vi "UI Main.vi"() -> ()   [LabVIEW 2013]
uses:
  controls/Control Configuration.ctl
  controls/Custom Controller Inputs.ctl
  controls/UI Data.ctl
  controls/All FPGA Configuration Values.ctl
  controls/FPGA State.ctl
  controls/Raw Values.ctl
  Globals/Global - All UI Loop Stop.vi
  Globals/Global - UI Stream and Variable Connections.vi
  Globals/Global - Configuration Options.vi
  support/User Event - Stop/User Event - Stop.lvlib
  support/Message Queue/Message Queue.lvlib
  <vilib>/Analysis/NI_AALBase.lvlib
panel:
  out "Connected? 2":bool=TRUE
  in  "Switch to Safe State":bool
  in  "Exit":bool
  out "System Status":string="\n5/12/2014 3:31:58 PM: UI Error -314220 - Read Single Element from Stream in UI - Read Stream from RT.vi->UI Main.vi\n5/12/2014 3:31:58 PM: UI Error -314220 - Read Single Element from Stream in UI - Read Stream from RT.vi->UI Main.vi\n5/12/2014 3:31:58 PM: UI Error -314220 - Read Single Element from Stream in UI - Read Stream from RT.vi->UI Main.vi\n5/12/2014 3:31:58 PM: UI Error -314220 - Read Single Element from Stream in UI - Read Stream from RT.vi->UI Main.vi\n5/12/2014 3:31:58 PM: UI Error -314220 - Read Single Element from Stream in UI - Read Stream from RT.vi->UI Main.vi\n5/12/2014 3:31:58 PM: UI Error -314220 - Read Single Element from Stream in UI - Read Stream from RT.vi->UI Main.vi\n5/12/2014 3:31:58 PM: UI Error -314220 - Read Single Element from Stream in UI - Read Stream from RT.vi->UI Main.vi\n5/12/2014 3:31:58 PM: UI Error -314220 - Read Single Element from Stream in UI - Read Stream from RT.vi->UI Main.vi\n5/12/2014 3:31:58 PM: UI Error -314220 - Read Single Element from Stream in UI - Read Stream from RT.vi->UI Main.vi\n5/12/2014 3:31:58 PM: UI Error -314220 - Read Single Element from Stream in UI - Read Stream from RT.vi->UI Main.vi\n5/12/2014 3:31:58 PM: UI Error -314220 - Read Single Element from Stream in UI - Read Stream from RT.vi->UI Main.vi\n5/12/2014 3:31:58 PM: UI Error -314220 - Read Single Element from Stream in UI - Read Stream from RT.vi->UI Main.vi\n5/12/2014 3:31:58 PM: UI Error -314220 - Read Single Element from Stream in UI - Read Stream from RT.vi->UI Main.vi\n5/12/2014 3:31:58 PM: UI Error -314220 - Read Single Element from Stream in UI - Read Stream from RT.vi->UI Main.vi\n5/12/2014 3:31:58 PM: UI Error -314220 - Read Single Element from Stream in UI - Read Stream from RT.vi->UI Main.vi\n5/12/2014 3:31:58 PM: UI Error -314220 - Read Single Element from Stream in UI - Read Stream from RT.vi->UI Main.vi\n5/12/2014 3:31:58 PM: UI Error -314220 - Write Single Element to Stream in UI Main.vi\n5/12/2014 3:31:36 PM: UI Error -314004 - Create Network Stream Writer Endpoint in UI - Initiate Connection.vi->UI Main.vi\n5/6/2014 11:02:04 PM: UI Error -314220 - Write Single Element to Stream in UI Main.vi"
  out "Current FPGA Control Mode":u16(ring)=2 items=["Safe State", "Manual", "Control (PID)"]
  in  "Settings Tab":T1(tab)
  in  "Control period (ticks)":u32=40000
  in  "Auto tare":bool
  in  "Channel 3 Setpoint":fxp<+/-,16,5>
  in  "Channel 2 Setpoint":fxp<+/-,16,5>
  in  "Channel 1 Setpoint":fxp<+/-,20,7>=7.0
  in  "Channel 0 Setpoint":fxp<+/-,20,7>
  in  "Update Control Configuration":bool
  in  "Control Configurations":T2[](array[typedef])=[{"PID Gains"={"proportional gain (Kc)"=55.0, "integral gain (Kc*Ts/Ti)"=0.0, "derivative gain (Kc*Td/Ts)"=0.0}, "Output Range"={"output high"=50.0, "output low"=-50.0}}, {"PID Gains"={"proportional gain (Kc)"=0.0, "integral gain (Kc*Ts/Ti)"=0.0, "derivative gain (Kc*Td/Ts)"=0.0}, "Output Range"={"output high"=10.0, "output low"=-10.0}}, {"PID Gains"={"proportional gain (Kc)"=0.0, "integral gain (Kc*Ts/Ti)"=0.0, "derivative gain (Kc*Td/Ts)"=0.0}, "Output Range"={"output high"=10.0, "output low"=-10.0}}, {"PID Gains"={"proportional gain (Kc)"=0.0, "integral gain (Kc*Ts/Ti)"=0.0, "derivative gain (Kc*Td/Ts)"=0.0}, "Output Range"={"output high"=10.0, "output low"=-10.0}}]
  in  "Run Control":bool
  in  "Stop Control":bool
  in  "Custom Controller Inputs":T3={"Other Controller Gains"={"Position Control Kp"=0.0, "Virtual Spring Constant (N/m)"=1000.0, "Offset weight (N)"=0.0, "Fthresh (N)"=1.0, "Var2"=0.0}}
  out "Offset (N)":fxp<+/-,16,8>
  in  "Channel 3 Manual Value":fxp<+/-,16,5>
  in  "Channel 2 Manual Value":fxp<+/-,16,5>
  in  "Channel 1 Manual Value":fxp<+/-,16,5>
  in  "Channel 0 Manual Value":fxp<+/-,16,5>
  in  "Run Manual":bool
  in  "Stop Manual":bool
  in  "Retain data":bool
  out "F std":dbl format="%#_4g"
  out "F avg":dbl format="%#_4g"
  in  "Clear Button":bool
  in  "Pause Button":bool
  in  "Save As Button":bool
  in  "Display frequency (Hz)":dbl=200.0 min=1.0 step=1.0
  out "Inputs (mV or V)":cluster{dbl[], dbl[]}[](graph)
  in  "Number of points":i32=1000 min=1 max=500000
  out "Force (N)":cluster{dbl[], dbl[]}(graph)
  out "V*":cluster{dbl[], dbl[]}(graph)
  out "Position (mm)":cluster{dbl[], dbl[]}(graph)
  out "Control loop frequency (Hz)":u32=40006
  out "Actual Loop Period (ticks)":u32=40006
  out "Largest Contiguous Memory (bytes)":dbl(graph)=60041648.0
  out "CPU Usage (%)":dbl(graph)=8.354955497028612
  out "Connected?":bool=TRUE
  in  "Connect to Controller":bool
  in  "Controller Address":string="169.254.66.100"
  # "LabVIEW FPGA Control on CompactRIO"
  # "Connection Settings"
  # "Force Command (N)"
  # "Position Command (mm)"
  # "Current Command (Testing)"
  # "Control period and setpoint changes are sent to the target automatically."
  # "Control Configuration changes are sent to the target when you click \"Update Control Configurations\"."
  # "Not used"
  # "Not used"
  # "Not used"
  # "F ="
  # "+/-"
  # "N"
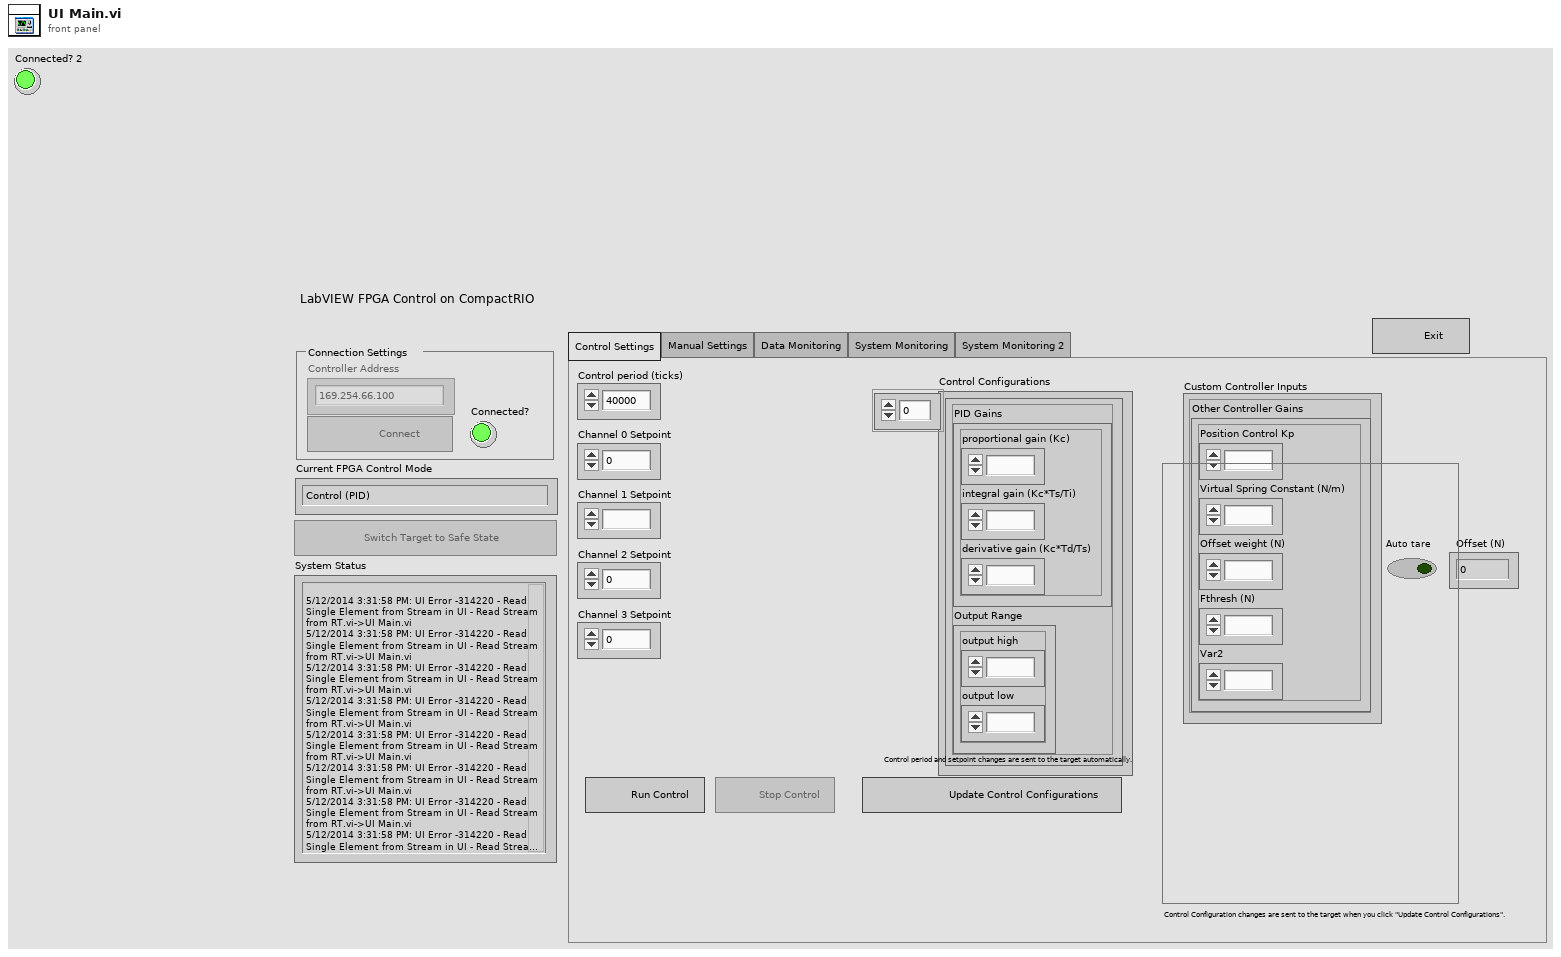
[diagram p1: front panel]
types:
  T1 = enum32{"Control Settings", "Manual Settings", "Data Monitoring", "System Monitoring", "System Monitoring 2"}
  T2 = typedef "Control Configuration.ctl" = cluster{"PID Gains":cluster{"proportional gain (Kc)":fxp<+/-,16,8>, "integral gain (Kc*Ts/Ti)":fxp<+/-,16,8>, "derivative gain (Kc*Td/Ts)":fxp<+/-,16,8>}, "Output Range":cluster{"output high":fxp<+/-,16,7>, "output low":fxp<+/-,16,7>}}
  T3 = typedef "Custom Controller Inputs.ctl" = cluster{"Other Controller Gains":cluster{"Position Control Kp":fxp<+/-,16,8>, "Virtual Spring Constant (N/m)":fxp<+,16,12>, "Offset weight (N)":fxp<+/-,16,8>, "Fthresh (N)":fxp<+/-,16,5>, "Var2":fxp<+/-,16,5>}}
  T4 = typedef "UI Data.ctl" = cluster{"Switch to Safe State Ref":refnum<vi>, "Run Manual Ref":refnum<vi>, "Stop Manual Ref":refnum<vi>, "Run Control Ref":refnum<vi>, "Stop Control Ref":refnum<vi>, "Update Control Configurations Ref":refnum<vi>, "Ch 0 Setpoint Ref":refnum<vi>, "Ch 1 Setpoint Ref":refnum<vi>, "Ch 2 Setpoint Ref":refnum<vi>, "Ch 3 Setpoint Ref":refnum<vi>, "Ch 0 Manual Ref":refnum<vi>, "Ch 1 Manual Ref":refnum<vi>, "Ch 2 Manual Ref":refnum<vi>, "Ch 3 Manual Ref":refnum<vi>, "Control Configurations Ref":refnum<vi>, "Custom Controller Cluster Ref":refnum<vi>, "Control period (ticks) Ref":refnum<vi>}
  T5 = typedef "Message Queue.lvlib/All Message Queues.ctl" = cluster{"UI":refnum<queue>}
  T6 = enum16{"open", "replace", "create", "open or create", "replace or create", "replace or create with confirmation"}
  T7 = cluster{"Channel 0 Setpoint":fxp<+/-,20,7>, "Channel 1 Setpoint":fxp<+/-,20,7>, "Channel 2 Setpoint":fxp<+/-,16,5>, "Channel 3 Setpoint":fxp<+/-,16,5>}
  T8 = cluster{"Channel 0 Manual Value":fxp<+/-,16,5>, "Channel 1 Manual Value":fxp<+/-,16,5>, "Channel 2 Manual Value":fxp<+/-,16,5>, "Channel 3 Manual Value":fxp<+/-,16,5>}
  T9 = typedef "Variable References.ctl" = cluster{"CPU Usage":refnum<k21>, "Contiguous Memory":refnum<k21>, "Input Values":refnum<k21>, "Output Values":refnum<k21>, "FPGA Mode":refnum<k21>, "Actual Loop Period":refnum<k21>}
  T10 = typedef "Raw Values.ctl" = cluster{"Channel 0":fxp<+/-,20,7>, "Channel 1":fxp<+/-,20,7>, "Channel 2":fxp<+/-,20,7>, "Channel 3":fxp<+/-,20,14>}
  T11 = cluster{"Channel 0":dbl, "Channel 1":dbl, "Channel 2":dbl, "Channel 3":dbl}
  T12 = cluster{"Message":string, "Message Data":variant}
  T13 = typedef "All FPGA Configuration Values.ctl" = cluster{"FPGA State":T14, "Manual Values":T10, "Setpoints":T10, "Control Configurations":T2[]}
  T14 = typedef "FPGA State.ctl" = enum16{"Safe State", "Manual", "Control (PID)"}
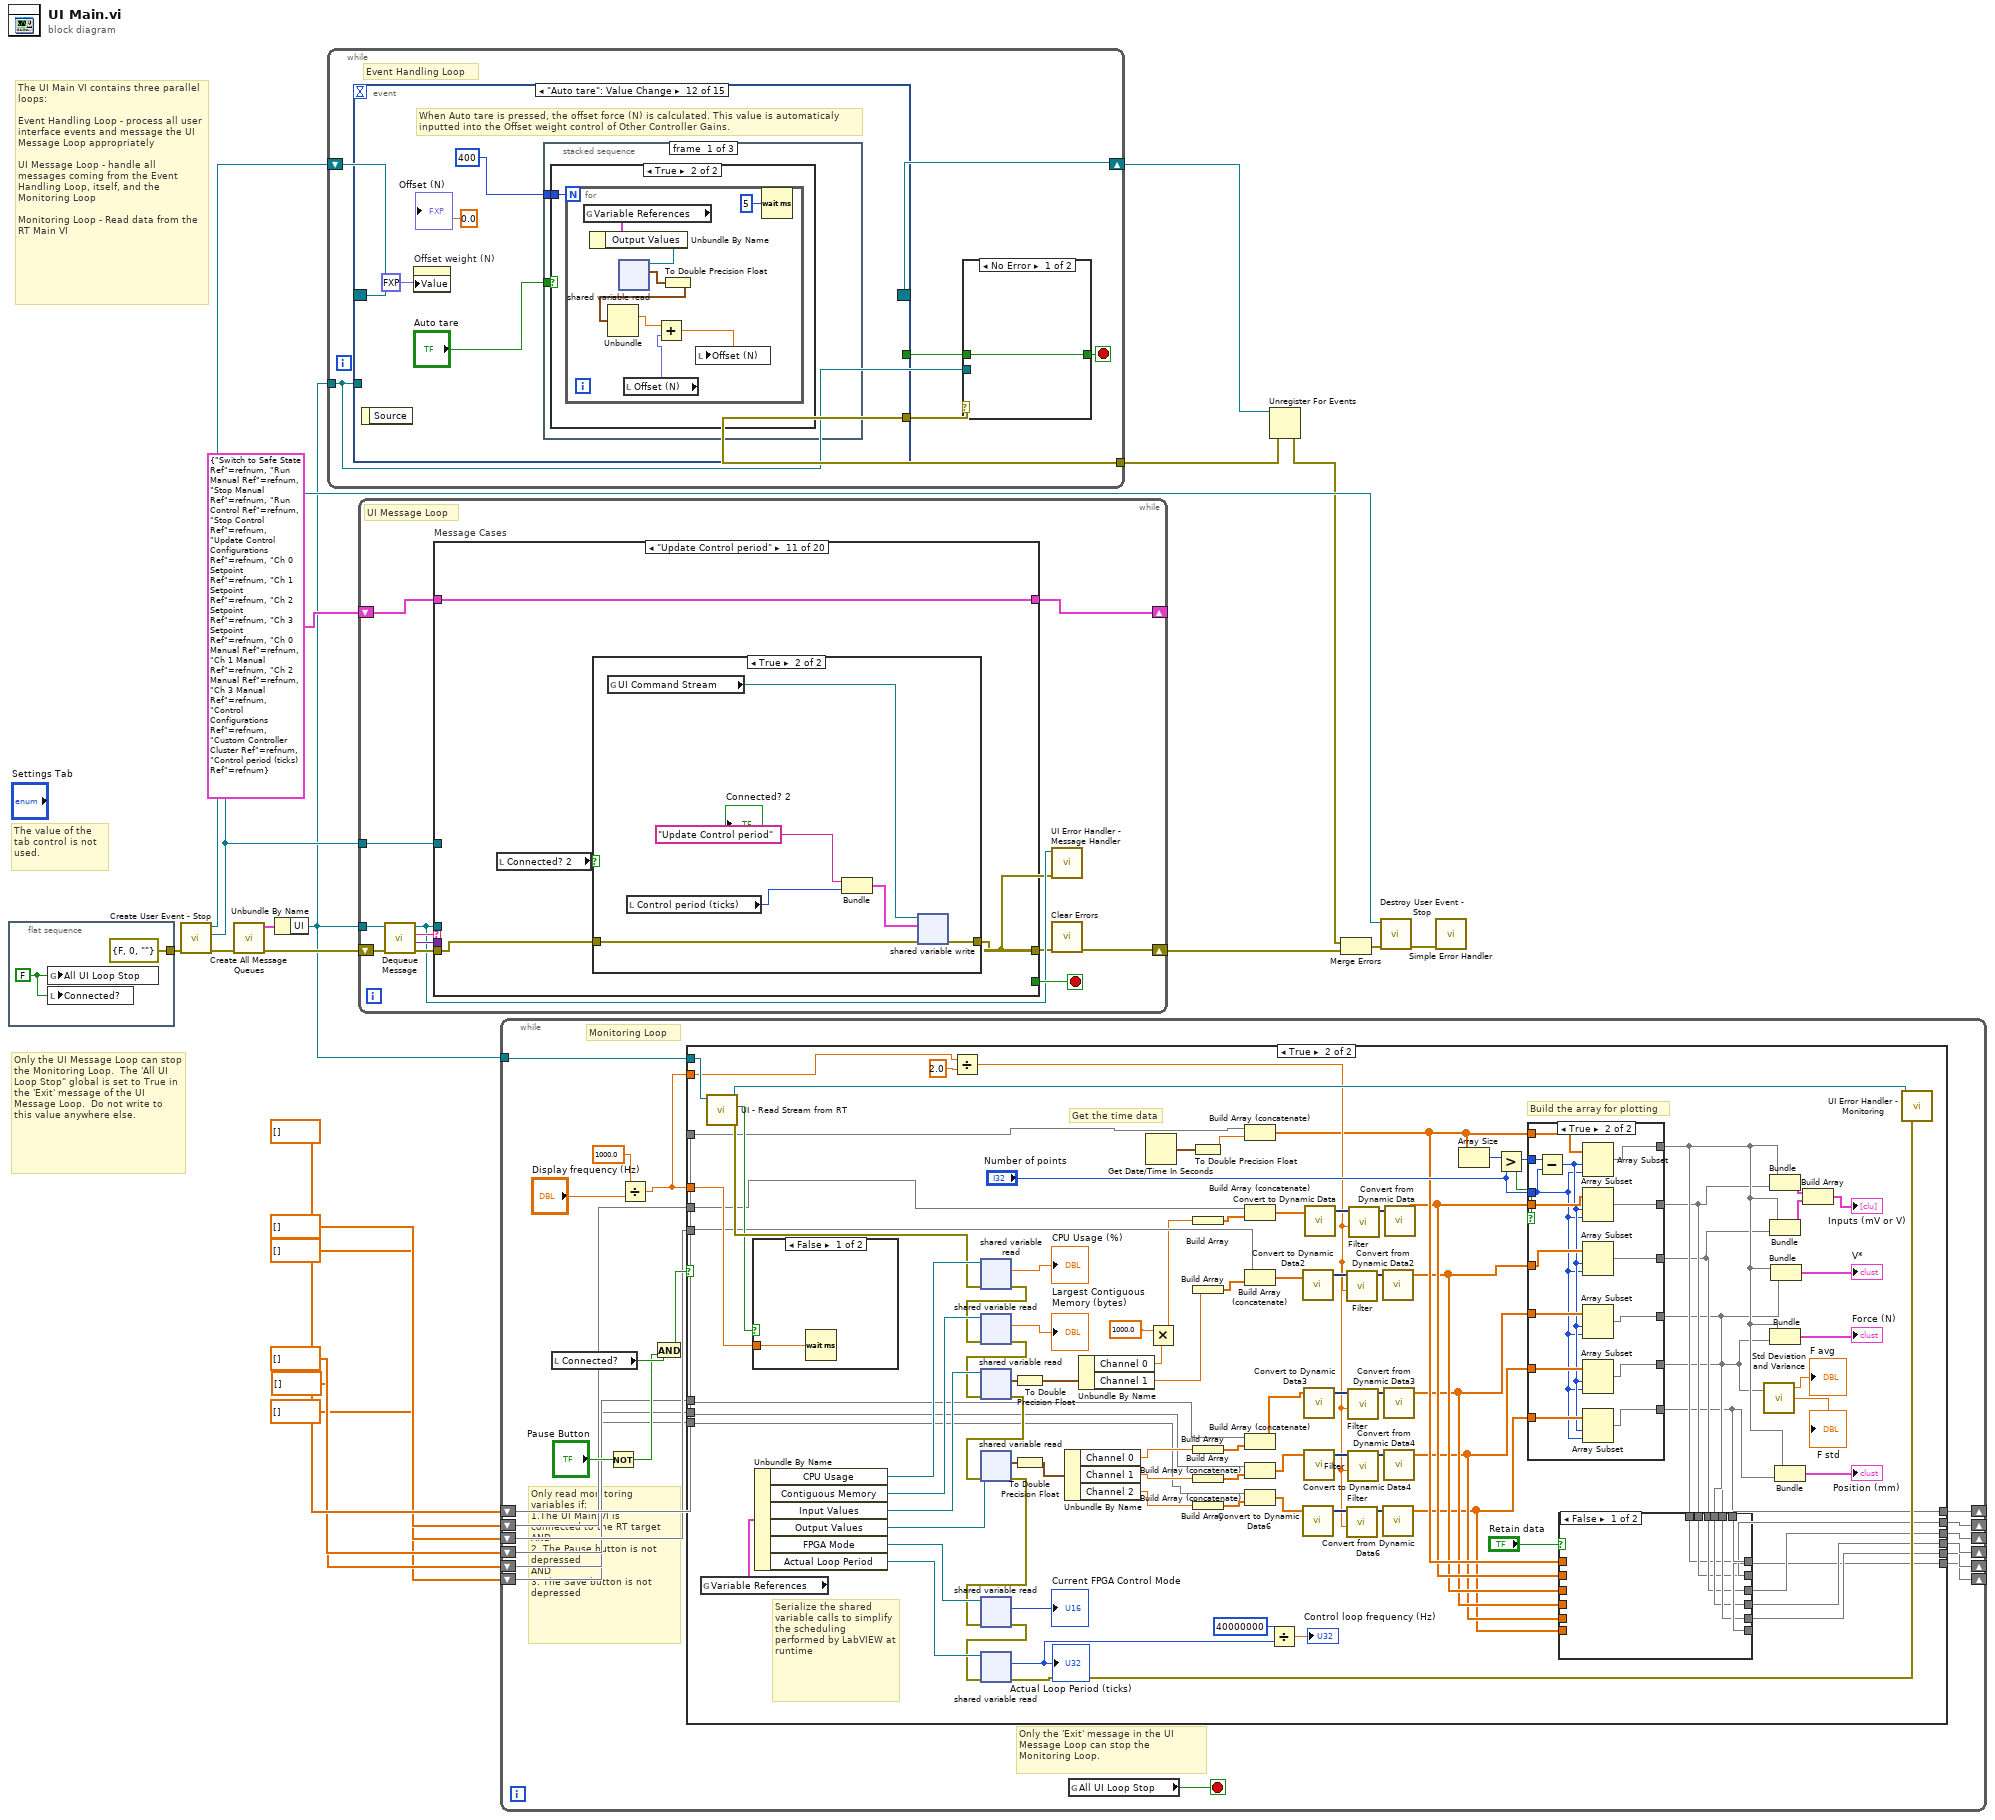
[diagram p0: block diagram]
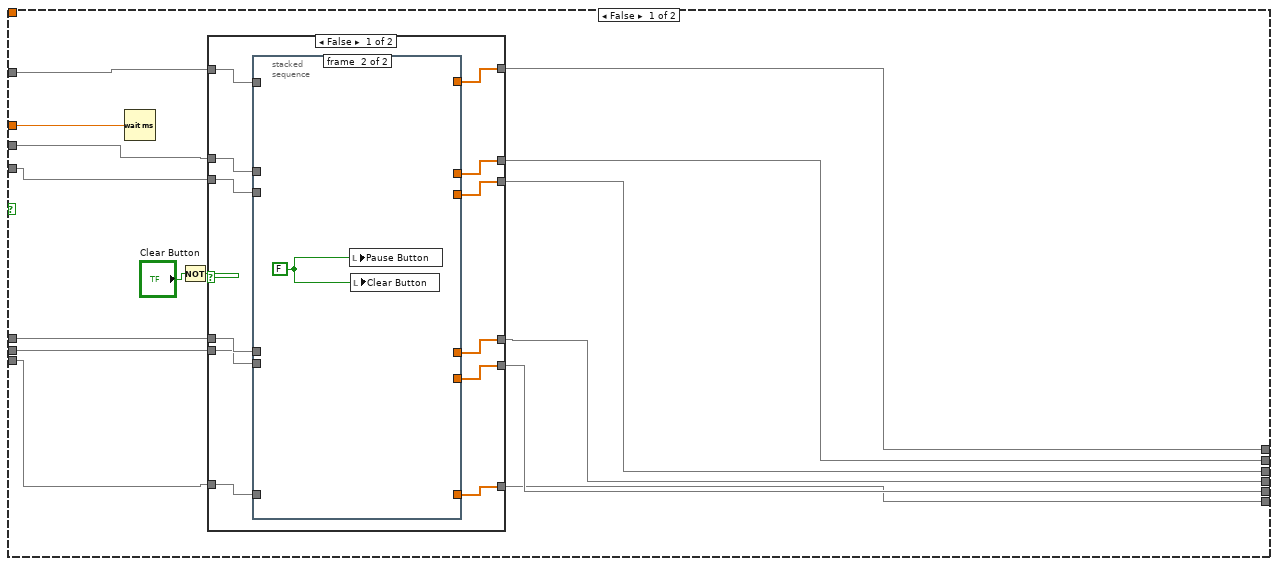
[diagram p2: hidden frame]
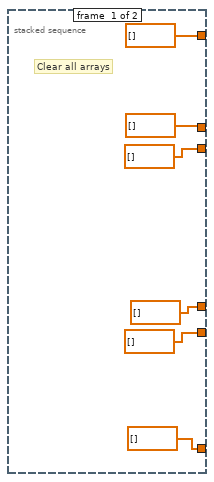
[diagram p3: hidden frame]
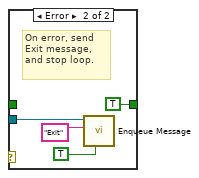
[diagram p8: hidden frame]
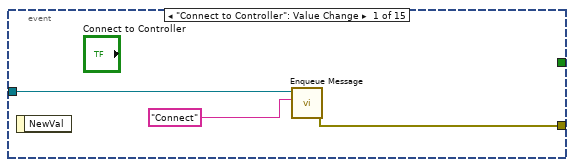
[diagram p9: hidden frame]
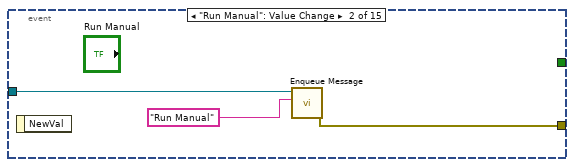
[diagram p10: hidden frame]
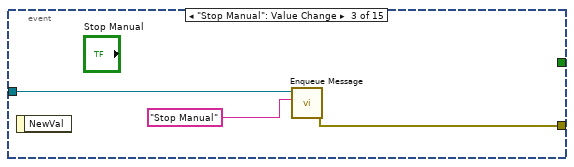
[diagram p11: hidden frame]
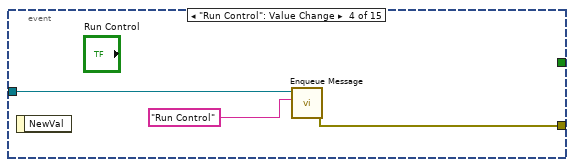
[diagram p12: hidden frame]
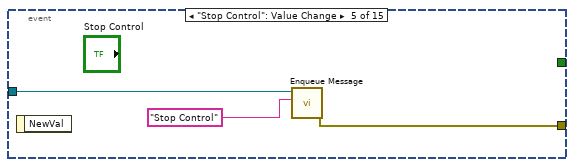
[diagram p13: hidden frame]
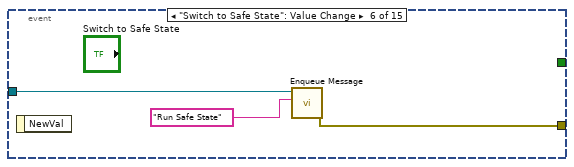
[diagram p14: hidden frame]
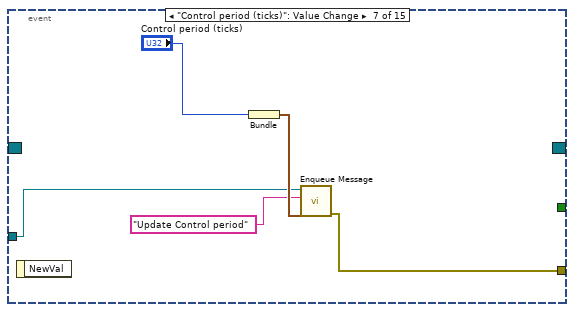
[diagram p15: hidden frame]
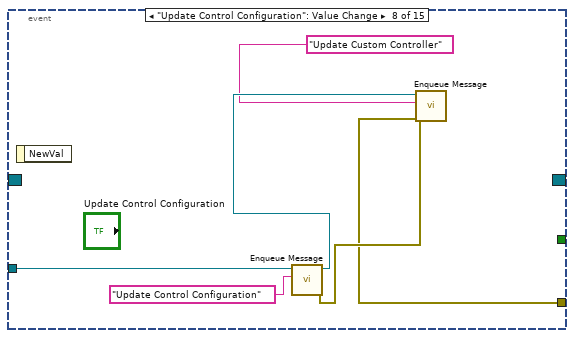
[diagram p16: hidden frame]
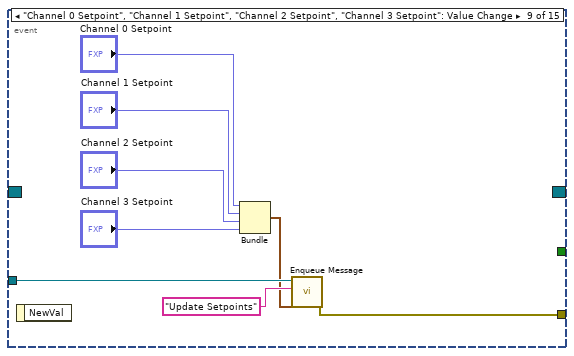
[diagram p17: hidden frame]
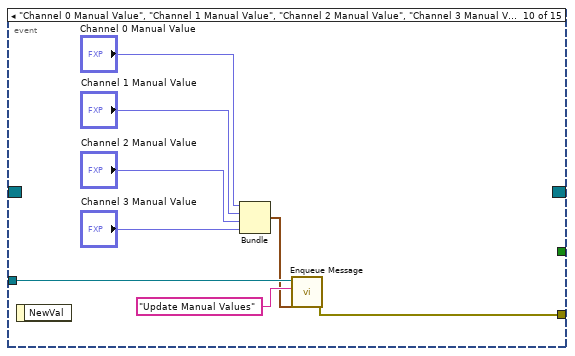
[diagram p18: hidden frame]
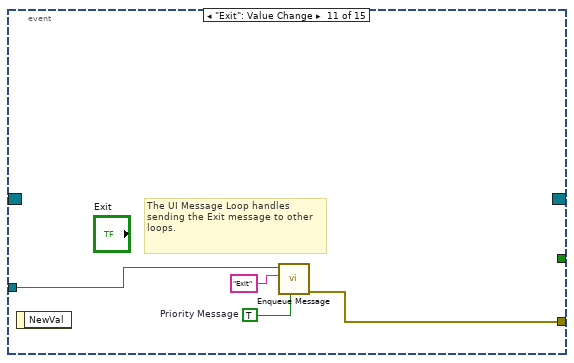
[diagram p19: hidden frame]
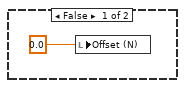
[diagram p20: hidden frame]
diagram:
  # "The UI Main VI contains three parallel loops:\n\nEvent Handling Loop - process all user interface events and message the UI Message Loop appropriately\n\nUI Message Loop - handle all messages coming from the Event Handling Loop, itself, and the Monitoring Loop\n\nMonitoring Loop - Read data from the RT Main VI"
  # "The value of the tab control is not used."
  # "Only the UI Message Loop can stop the Monitoring Loop.  The 'All UI Loop Stop\" global is set to True in the 'Exit' message of the UI Message Loop.  Do not write to this value anywhere else."
  n1 = flat-sequence {
    tunnel: [errorcluster {"status"=FALSE, "code"=0, "source"=""} ("error in (no error)")] -> w7
    frame #0 {
      w21 = FALSE
      n2 = global write "Global - All UI Loop Stop.vi" "All UI Loop Stop"(w21) -> ()
      n3 = local write "Connected?"(w21) -> ()
    }
  }
  n4 = call "Create User Event - Stop.vi"("error in (no error)"=w7) -> ("error out"=w15:errorcluster, "User Event - Stop"=w16:refnum<user-event>, "Stop Event Registration Refnum"=w17:refnum<event-registration>)  [unwired: 8 in]
  n5 = call "Create All Message Queues.vi"("error in (no error)"=w15) -> ("error out"=w13:errorcluster, "Message Queues out"=w14:T5)  [unwired: 9 in]
  n6 = Unbundle By Name(w14) -> ("UI"=w8:refnum<queue>)
  n7 = while {
    tunnel: w8 -> [w24]
    tunnel: [w26] -> w19
    shift-right: [w23] -> w11
    shift-left: w17 -> [w25]
    stop <- w27 stop-if-true
    # "Event Handling Loop"
    n8 = event shown="[11] \"Auto tare\": Value Change" {
      selector: w25 -> [_ _ _ _ _ _ _ _ _ _ _ _ _ _ _]
      dyn-events: [_ _ _ _ _ _ _ _ _ _ _ _ _ _ _] -> w23
      timeout: _ -> [_ _ _ _ _ _ _ _ _ _ _ _ _ _ _]
      tunnel: [_ _ _ _ _ _ _ _ _ _ _ _ TRUE ("Discard?") _ _] -> w28
      tunnel: w24 -> [w34 w37 w40 w43 w46 w49 w55 w62 w65 w74 w79 _ _ _ _]
      tunnel: [w36 w39 w42 w45 w48 w51 w52 w58 w64 w73 w82 _ _ _ _] -> w26
      event "Connect to Controller": Value Change {
        n9 = event-data() -> ()  [unwired: 1 in, 1 out]
        n10 = call "Enqueue Message.vi"("Message"="Connect", "Message Queue"=w34) -> ("error out"=w36:errorcluster)  [unwired: 8 in, 1 out]
      }
      event "Run Manual": Value Change {
        n11 = event-data() -> ()  [unwired: 1 in, 1 out]
        n12 = call "Enqueue Message.vi"("Message"="Run Manual", "Message Queue"=w37) -> ("error out"=w39:errorcluster)  [unwired: 8 in, 1 out]
      }
      event "Stop Manual": Value Change {
        n13 = event-data() -> ()  [unwired: 1 in, 1 out]
        n14 = call "Enqueue Message.vi"("Message"="Stop Manual", "Message Queue"=w40) -> ("error out"=w42:errorcluster)  [unwired: 8 in, 1 out]
      }
      event "Run Control": Value Change {
        n15 = event-data() -> ()  [unwired: 1 in, 1 out]
        n16 = call "Enqueue Message.vi"("Message"="Run Control", "Message Queue"=w43) -> ("error out"=w45:errorcluster)  [unwired: 8 in, 1 out]
      }
      event "Stop Control": Value Change {
        n17 = event-data() -> ()  [unwired: 1 in, 1 out]
        n18 = call "Enqueue Message.vi"("Message"="Stop Control", "Message Queue"=w46) -> ("error out"=w48:errorcluster)  [unwired: 8 in, 1 out]
      }
      event "Switch to Safe State": Value Change {
        n19 = event-data() -> ()  [unwired: 1 in, 1 out]
        n20 = call "Enqueue Message.vi"("Message"="Run Safe State", "Message Queue"=w49) -> ("error out"=w51:errorcluster)  [unwired: 8 in, 1 out]
      }
      event "Control period (ticks)": Value Change {
        n21 = event-data() -> ()  [unwired: 1 in, 1 out]
        n22 = Bundle("Control period (ticks)"="Control period (ticks)") -> (w56:cluster{"Control period (ticks)":u32})  [unwired: 1 in]
        n23 = call "Enqueue Message.vi"("Message Data"=w56, "Message"="Update Control period", "Message Queue"=w55) -> ("error out"=w52:errorcluster)  [unwired: 7 in, 1 out]
      }
      event "Update Control Configuration": Value Change {
        n24 = event-data() -> ()  [unwired: 1 in, 1 out]
        n25 = call "Enqueue Message.vi"("Message"="Update Control Configuration", "Message Queue"=w62) -> ("error out"=w59:errorcluster, "dup Message Queue"=w60:refnum<queue>)  [unwired: 8 in]
        n26 = call "Enqueue Message.vi"("error in (no error)"=w59, "Message"="Update Custom Controller", "Message Queue"=w60) -> ("error out"=w58:errorcluster)  [unwired: 7 in, 1 out]
      }
      event "Channel 0 Setpoint", "Channel 1 Setpoint", "Channel 2 Setpoint", "Channel 3 Setpoint": Value Change {
        n27 = event-data() -> ()  [unwired: 1 in, 1 out]
        n28 = Bundle("Channel 0 Setpoint"="Channel 0 Setpoint", "Channel 1 Setpoint"="Channel 1 Setpoint", "Channel 2 Setpoint"="Channel 2 Setpoint", "Channel 3 Setpoint"="Channel 3 Setpoint") -> (w63:T7)  [unwired: 1 in]
        n29 = call "Enqueue Message.vi"("Message Data"=w63, "Message"="Update Setpoints", "Message Queue"=w65) -> ("error out"=w64:errorcluster)  [unwired: 7 in, 1 out]
      }
      event "Channel 0 Manual Value", "Channel 1 Manual Value", "Channel 2 Manual Value", "Channel 3 Manual Value": Value Change {
        n30 = event-data() -> ()  [unwired: 1 in, 1 out]
        n31 = Bundle("Channel 0 Manual Value"="Channel 0 Manual Value", "Channel 1 Manual Value"="Channel 1 Manual Value", "Channel 2 Manual Value"="Channel 2 Manual Value", "Channel 3 Manual Value"="Channel 3 Manual Value") -> (w71:T8)  [unwired: 1 in]
        n32 = call "Enqueue Message.vi"("Message Data"=w71, "Message"="Update Manual Values", "Message Queue"=w74) -> ("error out"=w73:errorcluster)  [unwired: 7 in, 1 out]
      }
      event "Exit": Value Change {
        w80 = TRUE  # Priority Message
        # "The UI Message Loop handles sending the Exit message to other loops."
        n33 = event-data() -> ()  [unwired: 1 in, 1 out]
        n34 = call "Enqueue Message.vi"("Priority Message? (F)"=w80, "Message"="Exit", "Message Queue"=w79) -> ("error out"=w82:errorcluster)  [unwired: 7 in, 1 out]
      }
      event "Auto tare": Value Change {
        # "When Auto tare is pressed, the offset force (N) is calculated. This value is automaticaly \ninputted into the Offset weight control of Other Controller Gains."
        n35 = event-data() -> ()  [unwired: 1 in, 1 out]
        n36 = property on="Offset weight (N)" class="DigNum (strict)"("Value"=fxp<+/-,16,8> 0.0) -> ()  [unwired: 2 in, 2 out]
        n37 = stacked-sequence {
          tunnel: "Auto tare" -> [w88 _ _]
          tunnel: 400 -> [w87 w101 _]
          frame #0 {
            n38 = case shown="True" w88 {
              tunnel: w87 -> [_ w90]
              frame False {
                n39 = local write "Offset (N)"(0.0 ("Test")) -> ()
              }
              frame True {
                n40 = for {
                  N: w90 -> [_]
                  n41 = global read "Global - UI Stream and Variable Connections.vi" "Variable References"() -> (w94:T9)
                  n42 = Unbundle By Name(w94) -> ("Output Values"=w95:refnum<k21>)
                  n43 = shared-variable-read(w95) -> (w96:T10)  [unwired: 1 in, 3 out]
                  n44 = local read "Offset (N)"() -> (w93:fxp<+/-,16,8>)
                  n45 = To Double Precision Float(number=w96) -> (double precision float=w97:T11)
                  n46 = Unbundle(w97) -> ("Channel 1"=w91:dbl)  [unwired: 3 out]
                  n47 = Add(x=w91, y=w93) -> (x+y=w92:dbl)
                  n48 = local write "Offset (N)"(w92) -> ()
                  n49 = Wait (ms)(milliseconds to wait=u32 5) -> ()  [unwired: 1 out]
                }
              }
            }
          }
          frame #1 {
            n50 = local read "Offset (N)"() -> (w102:fxp<+/-,16,8>)
            n51 = To Double Precision Float(number=w101) -> (double precision float=w100:dbl)
            n52 = Divide(x=w102, y=w100) -> (x/y=w99:dbl)
            n53 = local write "Offset (N)"(w99) -> ()
          }
          frame #2 {
            n54 = local read "Offset (N)"() -> (w103:fxp<+/-,16,8>)
            n55 = property on="Offset weight (N)" class="DigNum (strict)"("Value"=w103) -> ()  [unwired: 2 in, 2 out]
          }
        }
        "Offset (N)" <- 0.0 ("Offset weight (N)")
      }
      event User Event {
        # "The Message Handling Loop processed an \"Exit\" message, which fired this event to stop the Event Handling Loop."
        n56 = event-data() -> ()  [unwired: 1 in, 1 out]
      }
      event "Save As Button": Value Change {
        # "When Save As is pressed, V*, Force, and Position are saved."
        n57 = event-data() -> ()  [unwired: 1 in, 1 out]
        n58 = stacked-sequence {
          frame #0 {
            n59 = local read "V*"() -> (w130:cluster{dbl[], dbl[]})
            n60 = local read "Force (N)"() -> (w129:cluster{dbl[], dbl[]})
            n61 = local read "Position (mm)"() -> (w128:cluster{dbl[], dbl[]})
            n62 = local write "Pause Button"(TRUE) -> ()
            n63 = Unbundle(w129) -> (w118:dbl[])  [unwired: 1 out]
            n64 = Unbundle(w130) -> (w116:dbl[], w119:dbl[])
            n65 = Unbundle(w128) -> (w117:dbl[])  [unwired: 1 out]
            n66 = Array Max & Min(array=w116) -> (min value=w114:dbl)  [unwired: 3 out]
            n67 = Subtract(x=w116, y=w114) -> (x-y=w115:dbl[])
            n68 = Build Array(w115, w119, w118, w117) -> (w122:dbl[][])
            n69 = Build Array("Time (s)" ("element"), "V* (V)" ("element"), "Force (N)" ("element"), "Position (mm)" ("element")) -> (w106:string[])
            n70 = Transpose 2D Array(2D array=w122) -> (transposed array=w120:dbl[][])
            n71 = Open/Create/Replace File(operation (0:open)=T6."replace or create") -> (refnum out=w123:refnum<file>, error out=w127:errorcluster)  [unwired: 5 in, 1 out]
            n72 = Array To Spreadsheet String(array=w106, 3:"%s") -> (spreadsheet string=w109:string)  [unwired: 1 in]
            n73 = Array To Spreadsheet String(array=w120, 3:"%g" ("format string")) -> (spreadsheet string=w108:string)  [unwired: 1 in]
            n74 = Concatenate Strings(w109, w108) -> (w107:string)
            n75 = Write to Text File(file (use dialog)=w123, text=w107, error in=w127) -> (refnum out=w125:refnum<file>, error out=w126:errorcluster)  [unwired: 2 out]
            n76 = Close File(refnum=w125, error in=w126) -> ()  [unwired: 2 out]
          }
          frame #1 {
            n77 = local write "Save As Button"(FALSE ("Pause Button")) -> ()
          }
        }
      }
      event "Clear Button": Value Change {
        # "When the Clear button is pressed, all data are erased."
        n78 = event-data() -> ()  [unwired: 1 in, 1 out]
        n79 = local write "Pause Button"(TRUE) -> ()
      }
    }
    n80 = case shown="No Error" w26 {
      tunnel: [w29 TRUE ("Discard?")] -> w27
      tunnel: w28 -> [w29 _]
      tunnel: w24 -> [_ w30]
      frame No Error {
      }
      frame Error {
        # "On error, send Exit message, and stop loop."
        n81 = call "Enqueue Message.vi"("Priority Message? (F)"=TRUE ("Discard?"), "Message"="Exit", "Message Queue"=w30) -> ()  [unwired: 7 in, 2 out]
      }
    }
  }
  n82 = while {
    tunnel: w8 -> [w139]
    tunnel: w16 -> [w144]
    shift-right: [w134] -> w20
    shift-left: w13 -> [w143]
    shift-right: [w137] -> _
    shift-left: T4 {"Switch to Safe State Ref"=refnum, "Run Manual Ref"=refnum, "Stop Manual Ref"=refnum, "Run Control Ref"=refnum, "Stop Control Ref"=refnum, "Update Control Configurations Ref"=refnum, "Ch 0 Setpoint Ref"=refnum, "Ch 1 Setpoint Ref"=refnum, "Ch 2 Setpoint Ref"=refnum, "Ch 3 Setpoint Ref"=refnum, "Ch 0 Manual Ref"=refnum, "Ch 1 Manual Ref"=refnum, "Ch 2 Manual Ref"=refnum, "Ch 3 Manual Ref"=refnum, "Control Configurations Ref"=refnum, "Custom Controller Cluster Ref"=refnum, "Control period (ticks) Ref"=refnum} ("Measurement UI Controls") -> [w138]
    stop <- w145 stop-if-true
    # "UI Message Loop"
    n83 = call "Dequeue Message.vi"("error in (no error)"=w143, "Message Queue"=w139) -> ("error out"=w142:errorcluster, "Message Data"=w140:variant, "Message"=w141:string, "dup Message Queue"=w136:refnum<queue>)  [unwired: 6 in]
    n84 = case "Message Cases" shown="\"Update Control period\"" w141 {
      selector: w141 -> [_ _ _ _ _ _ _ _ _ w274 _ _ _ w328 _ w378 _ _ _ w439]
      tunnel: w136 -> [w147 w155 _ _ w214 _ w232 _ w250 w275 _ _ _ _ _ w382 _ w424 _ _]
      tunnel: w142 -> [w149 w173 w195 w198 w219 w230 w234 w239 w270 w277 w294 w306 w317 w329 w349 w392 w413 w429 w434 _]
      tunnel: [w148 w156 w195 w198 w213 w230 w233 w238 w253 w276 w293 w305 w316 w330 w348 w393 w411 w430 w433 w437] -> w135
      tunnel: [_ _ _ _ _ _ _ _ _ _ _ _ _ _ _ _ _ TRUE _ _] -> w145
      tunnel: w140 -> [_ _ _ _ _ _ _ _ w268 _ _ _ _ w327 w347 w390 w410 _ _ _]
      tunnel: w144 -> [_ _ _ _ _ _ _ _ _ _ _ _ _ _ _ _ _ w428 _ _]
      tunnel: w138 -> [w150 w172 w194 w209 w218 w229 w236 w240 w265 w278 w296 w307 w318 w331 w346 w394 w412 w426 w432 w435]
      tunnel: [w150 w171 w194 w209 w218 w229 w236 w240 w265 w278 w296 w307 w318 w331 w346 w394 w412 w426 w432 w435] -> w137
      frame "Initialize" {
        # "Initialize - Send 'Initialize UI Refs' message to get the UI references bundled and initialized appropriately."
        n85 = call "Enqueue Message.vi"("error in (no error)"=w149, "Message"="Initialize UI Refs", "Message Queue"=w147) -> ("error out"=w148:errorcluster)  [unwired: 7 in, 1 out]
      }
      frame "Initialize UI Refs" {
        # "Send a message to disable them all, since there is no connection at the start."
        # "Initialize UI Refs - Bundle up a cluster of references of all UI elements that are programmatically manipulated."
        n86 = control-ref of="Switch to Safe State"() -> (w170:refnum<vi>)
        n87 = control-ref of="Run Manual"() -> (w169:refnum<vi>)
        n88 = control-ref of="Stop Manual"() -> (w168:refnum<vi>)
        n89 = control-ref of="Run Control"() -> (w167:refnum<vi>)
        n90 = control-ref of="Stop Control"() -> (w166:refnum<vi>)
        n91 = control-ref of="Update Control Configuration"() -> (w165:refnum<vi>)
        n92 = control-ref of="Control period (ticks)"() -> (w151:refnum<vi>)
        n93 = control-ref of="Other Controller Gains"() -> (w152:refnum<vi>)
        n94 = control-ref of="Custom Controller Inputs"() -> ()  [unwired: 1 out]
        n95 = control-ref of="Channel 0 Setpoint"() -> (w164:refnum<vi>)
        n96 = control-ref of="Channel 1 Setpoint"() -> (w163:refnum<vi>)
        n97 = control-ref of="Channel 2 Setpoint"() -> (w162:refnum<vi>)
        n98 = control-ref of="Channel 3 Setpoint"() -> (w161:refnum<vi>)
        n99 = control-ref of="Channel 0 Manual Value"() -> (w160:refnum<vi>)
        n100 = control-ref of="Channel 1 Manual Value"() -> (w159:refnum<vi>)
        n101 = control-ref of="Channel 2 Manual Value"() -> (w158:refnum<vi>)
        n102 = control-ref of="Channel 3 Manual Value"() -> (w157:refnum<vi>)
        n103 = control-ref of="Control Configurations"() -> (w153:refnum<vi>)
        n104 = call "Enqueue Message.vi"("error in (no error)"=w173, "Message"="Disable Controls", "Message Queue"=w155) -> ("error out"=w156:errorcluster)  [unwired: 7 in, 1 out]
        n105 = Bundle By Name(cluster=w172, "Switch to Safe State Ref"=w170, "Run Manual Ref"=w169, "Stop Manual Ref"=w168, "Run Control Ref"=w167, "Stop Control Ref"=w166, "Update Control Configurations Ref"=w165, "Ch 0 Setpoint Ref"=w164, "Ch 1 Setpoint Ref"=w163, "Ch 2 Setpoint Ref"=w162, "Ch 3 Setpoint Ref"=w161, "Ch 0 Manual Ref"=w160, "Ch 1 Manual Ref"=w159, "Ch 2 Manual Ref"=w158, "Ch 3 Manual Ref"=w157, "Control Configurations Ref"=w153, "Custom Controller Cluster Ref"=w152, "Control period (ticks) Ref"=w151) -> (w171:T4)
      }
      frame "Disable Controls" {
        w176 = 0
        # "With the control options disabled, the only thing the user can do is Connect. Make sure the IP address string and connect button are enabled."
        # "Disable All Controls - Set all controls in the UI Refs cluster to \"Disabled and Grayed Out\"."
        n106 = Unbundle(w194) -> ("Switch to Safe State Ref"=w193:refnum<vi>, "Run Manual Ref"=w192:refnum<vi>, "Stop Manual Ref"=w191:refnum<vi>, "Run Control Ref"=w190:refnum<vi>, "Stop Control Ref"=w189:refnum<vi>, "Update Control Configurations Ref"=w188:refnum<vi>, "Ch 0 Setpoint Ref"=w187:refnum<vi>, "Ch 1 Setpoint Ref"=w186:refnum<vi>, "Ch 2 Setpoint Ref"=w185:refnum<vi>, "Ch 3 Setpoint Ref"=w184:refnum<vi>, "Ch 0 Manual Ref"=w183:refnum<vi>, "Ch 1 Manual Ref"=w182:refnum<vi>, "Ch 2 Manual Ref"=w181:refnum<vi>, "Ch 3 Manual Ref"=w180:refnum<vi>, "Control Configurations Ref"=w179:refnum<vi>, "Custom Controller Cluster Ref"=w175:refnum<vi>, "Control period (ticks) Ref"=w174:refnum<vi>)
        n107 = Build Array(w193, w192, w191, w190, w189, w188, w187, w186, w185, w184, w183, w182, w181, w180, w179, w175, w174) -> (w178:refnum<vi>[])
        n108 = call "Set Enable State on Multiple Controls.vi"("Enable?"=FALSE, "Controls"=w178) -> ()  [unwired: 10 in]
        n109 = property on="Controller Address" class="Str"("DisabledEnum"=w176) -> ()  [unwired: 2 in, 2 out]
        n110 = property on="Connect to Controller" class="Bool"("DisabledEnum"=w176) -> ()  [unwired: 2 in, 2 out]
      }
      frame "Enable Configuration Controls" {
        w210 = 2
        # "Once connected, the user shouldn't be able to change the connection settings unless he gets disconnected."
        # "Enable Configuration Controls - After successful connection, ensure appropriate controls are enabled."
        n111 = Unbundle By Name(w209) -> ("Update Control Configurations Ref"=w208:refnum<vi>, "Ch 0 Setpoint Ref"=w207:refnum<vi>, "Ch 1 Setpoint Ref"=w206:refnum<vi>, "Ch 2 Setpoint Ref"=w205:refnum<vi>, "Ch 3 Setpoint Ref"=w204:refnum<vi>, "Ch 0 Manual Ref"=w203:refnum<vi>, "Ch 1 Manual Ref"=w202:refnum<vi>, "Ch 2 Manual Ref"=w201:refnum<vi>, "Ch 3 Manual Ref"=w200:refnum<vi>, "Control Configurations Ref"=w199:refnum<vi>, "Custom Controller Cluster Ref"=w197:refnum<vi>, "Control period (ticks) Ref"=w196:refnum<vi>)
        n112 = Build Array(w208, w207, w206, w205, w204, w203, w202, w201, w200, w199, w197, w196) -> (w212:refnum<vi>[])
        n113 = call "Set Enable State on Multiple Controls.vi"("Enable?"=TRUE, "Controls"=w212) -> ()  [unwired: 10 in]
        n114 = property on="Controller Address" class="Str"("DisabledEnum"=w210) -> ()  [unwired: 2 in, 2 out]
        n115 = property on="Connect to Controller" class="Bool"("DisabledEnum"=w210) -> ()  [unwired: 2 in, 2 out]
      }
      frame "Connect" {
        # "Connect - Attempt to connect to both streams, and the variables, on the RT target."
        n116 = call "UI - Initiate Connection.vi"("error in (no error)"=w219, "Controller Address"="Controller Address", "Message Queue"=w214) -> ("error out"=w216:errorcluster, "Connected?"=w215:bool)  [unwired: 7 in]
        "Connected?" <- w215
        n117 = case shown="True" w215 {
          tunnel: w216 -> [w220 w224]
          tunnel: w214 -> [_ w223]
          tunnel: [w220 w222] -> w213
          frame False {
          }
          frame True {
            n118 = call "Enqueue Message.vi"("error in (no error)"=w224, "Message"="Enable Configuration Controls", "Message Queue"=w223) -> ("error out"=w222:errorcluster)  [unwired: 7 in, 1 out]
          }
        }
      }
      frame "Close Connections" {
        # "Close Connections - Close the connections shared with the Monitoring Loop."
        n119 = global read "Global - UI Stream and Variable Connections.vi" "UI Command Stream"() -> (w228:refnum<k21>)
        n120 = global read "Global - UI Stream and Variable Connections.vi" "RT Message Stream"() -> (w227:refnum<k21>)
        n121 = global read "Global - UI Stream and Variable Connections.vi" "Variable References"() -> (w226:T9)
        n122 = local write "Connected?"(FALSE ("Connected?")) -> ()
        n123 = Destroy Stream Endpoint(11:w228) -> ()  [unwired: 1 in, 1 out]
        n124 = Destroy Stream Endpoint(11:w227) -> ()  [unwired: 1 in, 1 out]
        n125 = call "Close Variable Connections.vi"("Variable References"=w226) -> ()  [unwired: 11 in]
      }
      frame "Disconnect UI" {
        # "Disconnect UI - Something has gone wrong with the connection. Reinitialize the UI to its disconnected state."
        n126 = local write "Connected?"(FALSE ("Connected?")) -> ()
        n127 = call "Enqueue Message.vi"("error in (no error)"=w234, "Message"="Disable Controls", "Message Queue"=w232) -> ("error out"=w233:errorcluster)  [unwired: 7 in, 1 out]
      }
      frame "Get Settings from FPGA" {
        # "Get Settings from FPGA - Send a command to the RT to retrieve all current FPGA Main VI parameter values and send them back to the UI."
        n128 = local read "Connected?"() -> (w237:bool)
        n129 = case shown="True" w237 {
          tunnel: w239 -> [w241 w245]
          tunnel: [w241 w244] -> w238
          frame False {
            # "Don't bother trying to send a message to the RT system if UI Main VI isn't even connected"
          }
          frame True {
            n130 = global read "Global - UI Stream and Variable Connections.vi" "UI Command Stream"() -> (w242:refnum<k21>)
            n131 = shared-variable-write(w242, w245, T12 {"Message"="Send FPGA Configuration to UI", "Message Data"=variant} ("data in")) -> (w244:errorcluster)  [unwired: 1 in, 2 out]
          }
        }
      }
      frame "Initial UI Values" {
        # "Initial UI Values - These are the current values of the FPGA Main VI's R/W controls. They are used to initialize the panel of UI Main VI upon successful connection to the RT target."
        # "Set values of all manual and setpoint controls via reference."
        n132 = Variant To Data(error in=w270, type=T13 {"FPGA State"=enum."Safe State", "Manual Values"={"Channel 0"=0.0, "Channel 1"=0.0, "Channel 2"=0.0, "Channel 3"=0.0}, "Setpoints"={"Channel 0"=0.0, "Channel 1"=0.0, "Channel 2"=0.0, "Channel 3"=0.0}, "Control Configurations"=[]} ("All FPGA Configuration Values"), Variant=w268) -> (data=w266:T13, error out=w269:errorcluster)
        n133 = Unbundle By Name(w265) -> ("Ch 0 Setpoint Ref"=w264:refnum<vi>, "Ch 1 Setpoint Ref"=w263:refnum<vi>, "Ch 2 Setpoint Ref"=w262:refnum<vi>, "Ch 3 Setpoint Ref"=w261:refnum<vi>, "Ch 0 Manual Ref"=w260:refnum<vi>, "Ch 1 Manual Ref"=w259:refnum<vi>, "Ch 2 Manual Ref"=w258:refnum<vi>, "Ch 3 Manual Ref"=w257:refnum<vi>)
        n134 = Unbundle By Name(w266) -> ("Setpoints"=w248:T10, "Manual Values"=w246:T10, "Control Configurations"=w254:T2[], "FPGA State"=w251:T14)
        n135 = Build Array(w264, w263, w262, w261, w260, w259, w258, w257) -> (w256:refnum<vi>[])
        n136 = To Variant(anything=w246) -> (Variant=w247:variant)
        n137 = To Variant(anything=w248) -> (Variant=w249:variant)
        n138 = local write "Current FPGA Control Mode"(w251) -> ()
        n139 = Build Array(w249, w247) -> (w255:variant[])
        n140 = local write "Control Configurations"(w254) -> ()
        n141 = for {
          tunnel: w256 -> [w272] mode=indexing
          tunnel: w255 -> [w271] mode=indexing
          n142 = property class="DigNum"(reference=w272, "Value"=w271) -> ()  [unwired: 1 in, 2 out]
        }
        n143 = call "Enqueue Message.vi"("error in (no error)"=w269, "Message Data"=w251, "Message"="Update Display Mode", "Message Queue"=w250) -> ("error out"=w253:errorcluster)  [unwired: 6 in, 1 out]
      }
      frame "Run Control", "Run Manual", "Run Safe State", "Stop Control", "Stop Manual" {
        # "Run/Stop buttons - Send a command to switch the FPGA into the appropriate state. Send a message to update this UI to reflect the new state."
        n144 = local read "Connected?"() -> (w273:bool)
        n145 = case shown="True" w273 {
          tunnel: w277 -> [w279 w289]
          tunnel: [w279 w285] -> w276
          tunnel: w275 -> [_ w284]
          tunnel: w274 -> [_ w283]
          frame False {
            # "Don't bother trying to send a message to the RT system if UI Main VI isn't even connected"
          }
          frame True {
            # "Run Manual and Run Control switch into their respective states. Anything else switches to Safe State."
            n146 = case shown="\"Run Control\"" w283 {
              tunnel: [FPGA_State."Safe State" ("FPGA State") FPGA_State."Control (PID)" ("FPGA State") FPGA_State."Manual" ("FPGA State")] -> w280
              frame "Safe State", "Stop Control", "Stop Manual", Default {
              }
              frame "Run Control" {
              }
              frame "Run Manual" {
              }
            }
            n147 = global read "Global - UI Stream and Variable Connections.vi" "UI Command Stream"() -> (w281:refnum<k21>)
            n148 = Bundle("Update FPGA State", "FPGA State"=w280) -> (w286:cluster{string, "FPGA State":T14})  [unwired: 1 in]
            n149 = shared-variable-write(w281, w289, w286) -> (w288:errorcluster)  [unwired: 1 in, 2 out]
            n150 = call "Enqueue Message.vi"("error in (no error)"=w288, "Message Data"=w280, "Message"="Update Display Mode", "Message Queue"=w284) -> ("error out"=w285:errorcluster)  [unwired: 6 in, 1 out]
          }
        }
      }
      frame "Update Control period" {
        n151 = local read "Connected? 2"() -> (w295:bool)
        n152 = case shown="True" w295 {
          tunnel: w294 -> [w297 w303]
          tunnel: [w297 w302] -> w293
          frame False {
            # "Don't bother trying to send a message to the RT system if UI Main VI isn't even connected"
          }
          frame True {
            n153 = global read "Global - UI Stream and Variable Connections.vi" "UI Command Stream"() -> (w299:refnum<k21>)
            n154 = local read "Control period (ticks)"() -> (w298:u32)
            n155 = Bundle("Update Control period", "Control period (ticks)"=w298) -> (w300:cluster{string, "Control period (ticks)":u32})  [unwired: 1 in]
            n156 = shared-variable-write(w299, w303, w300) -> (w302:errorcluster)  [unwired: 1 in, 2 out]
          }
        }
      }
      frame "Update Control Configuration" {
        # "Update Control Configuration - Send all control configurations to RT to be sent down to the FPGA."
        n157 = local read "Connected?"() -> (w304:bool)
        n158 = case shown="True" w304 {
          tunnel: w306 -> [w308 w314]
          tunnel: [w308 w313] -> w305
          frame False {
            # "Don't bother trying to send a message to the RT system if UI Main VI isn't even connected"
          }
          frame True {
            n159 = global read "Global - UI Stream and Variable Connections.vi" "UI Command Stream"() -> (w309:refnum<k21>)
            n160 = Bundle("Update Control Configurations", "Control Configurations"="Control Configurations") -> (w311:cluster{string, "Control Configurations":T2[]})  [unwired: 1 in]
            n161 = shared-variable-write(w309, w314, w311) -> (w313:errorcluster)  [unwired: 1 in, 2 out]
          }
        }
      }
      frame "Update Custom Controller" {
        # "Update Control Configuration - Send all control configurations to RT to be sent down to the FPGA."
        n162 = local read "Connected?"() -> (w315:bool)
        n163 = case shown="True" w315 {
          tunnel: w317 -> [w319 w325]
          tunnel: [w319 w324] -> w316
          frame False {
            # "Don't bother trying to send a message to the RT system if UI Main VI isn't even connected"
          }
          frame True {
            n164 = global read "Global - UI Stream and Variable Connections.vi" "UI Command Stream"() -> (w321:refnum<k21>)
            n165 = Bundle("Update Custom Controller", "Custom Controller Inputs"="Custom Controller Inputs") -> (w322:cluster{string, "Custom Controller Inputs":T3})  [unwired: 1 in]
            n166 = shared-variable-write(w321, w325, w322) -> (w324:errorcluster)  [unwired: 1 in, 2 out]
          }
        }
      }
      frame "Update Manual Values", "Update Setpoints" {
        # "Update Manual Values/Setpoints - Send all manual values/setpoints to RT to be sent down to the FPGA."
        n167 = local read "Connected?"() -> (w326:bool)
        n168 = case shown="True" w326 {
          tunnel: [w332 w338] -> w330
          tunnel: w329 -> [w332 w336]
          tunnel: w328 -> [_ w335]
          tunnel: w327 -> [_ w334]
          frame False {
            # "Don't bother trying to send a message to the RT system if UI Main VI isn't even connected"
          }
          frame True {
            n169 = global read "Global - UI Stream and Variable Connections.vi" "UI Command Stream"() -> (w333:refnum<k21>)
            n170 = Bundle(w335, "Message Data"=w334) -> (w337:cluster{string, "Message Data":variant})  [unwired: 1 in]
            n171 = shared-variable-write(w333, w336, w337) -> (w338:errorcluster)  [unwired: 1 in, 2 out]
          }
        }
      }
      frame "Update Display Mode" {
        # "Update Display Mode - Enable/Disable Controls appropriately for the new display mode."
        n172 = Variant To Data(error in=w349, type=FPGA_State."Safe State" ("FPGA State"), Variant=w347) -> (data=w345:T14, error out=w348:errorcluster)
        n173 = Unbundle By Name(w346) -> ("Switch to Safe State Ref"=w344:refnum<vi>, "Run Manual Ref"=w343:refnum<vi>, "Stop Manual Ref"=w342:refnum<vi>, "Run Control Ref"=w341:refnum<vi>, "Stop Control Ref"=w340:refnum<vi>)
        n174 = case shown="\"Control (PID)\"" w345 {
          tunnel: w344 -> [w354 w363 w370]
          tunnel: w343 -> [w350 w362 w372]
          tunnel: w342 -> [w353 w361 w369]
          tunnel: w341 -> [w352 w359 w371]
          tunnel: w340 -> [w351 w360 w368]
          frame "Control (PID)" {
            n175 = Build Array "Controls to Enable"(w354, w351, w350) -> (w358:refnum<vi>[])
            n176 = Build Array "Controls to Disable"(w353, w352) -> (w356:refnum<vi>[])
            n177 = call "Set Enable State on Multiple Controls.vi"("Enable?"=FALSE, "Controls"=w356) -> ()  [unwired: 10 in]
            n178 = call "Set Enable State on Multiple Controls.vi"("Enable?"=TRUE, "Controls"=w358) -> ()  [unwired: 10 in]
          }
          frame "Manual" {
            n179 = Build Array "Controls to Enable"(w363, w361, w359) -> (w367:refnum<vi>[])
            n180 = Build Array "Controls to Disable"(w362, w360) -> (w365:refnum<vi>[])
            n181 = call "Set Enable State on Multiple Controls.vi"("Enable?"=FALSE, "Controls"=w365) -> ()  [unwired: 10 in]
            n182 = call "Set Enable State on Multiple Controls.vi"("Enable?"=TRUE, "Controls"=w367) -> ()  [unwired: 10 in]
          }
          frame "Safe State" {
            # "This frame runs when FPGA is in Safe State. Only enable the two run buttons."
            n183 = Build Array "Controls to Enable"(w372, w371) -> (w376:refnum<vi>[])
            n184 = Build Array "Controls to Disable"(w370, w369, w368) -> (w374:refnum<vi>[])
            n185 = call "Set Enable State on Multiple Controls.vi"("Enable?"=FALSE, "Controls"=w374) -> ()  [unwired: 10 in]
            n186 = call "Set Enable State on Multiple Controls.vi"("Enable?"=TRUE, "Controls"=w376) -> ()  [unwired: 10 in]
          }
        }
      }
      frame "Critical Error", "Log-Only Error", "Non-Critical Error", "RT Error" {
        # "Error - Display message in status indicator on panel.  If it's a critical error, shut down this VI with an 'Exit' message."
        n187 = case shown="Default" w378 {
          selector: w378 -> [_ w396]
          tunnel: ["UI Error" w396] -> w377
          frame Default {
          }
          frame "RT Error" {
          }
        }
        n188 = Variant To Data(error in=w392, type=errorcluster {"status"=FALSE, "code"=0, "source"=""} ("error constant"), Variant=w390) -> (data=w385:errorcluster, error out=w391:errorcluster)
        n189 = Unbundle By Name(w385) -> ("code"=w384:i32, "source"=w388:string)
        n190 = Format Date/Time String() -> (date/time string=w387:string)  [unwired: 3 in]
        n191 = Format Into String(format string="\n%s: %s %d - %s", w387, w377, w384, w388) -> (resulting string=w379:string)  [unwired: 2 in, 1 out]
        n192 = call "Enqueue Message.vi"("error in (no error)"=w391, "Message Data"=w379, "Message"="Update System Status", "Message Queue"=w382) -> ("error out"=w383:errorcluster, "dup Message Queue"=w381:refnum<queue>)  [unwired: 6 in]
        n193 = case shown="Default" w378 {
          tunnel: w383 -> [w397 w401]
          tunnel: w381 -> [_ w399]
          tunnel: [w397 w400] -> w393
          frame Default {
          }
          frame "Critical Error" {
            n194 = call "Enqueue Message.vi"("error in (no error)"=w401, "Message"="Exit", "Message Queue"=w399) -> ("error out"=w400:errorcluster)  [unwired: 7 in, 1 out]
          }
        }
      }
      frame "Update System Status" {
        # "Code Recommended - The code below ensures that the System Status string value does not become too large.  It uses the same maximum size as the RT error log to determine whether or not to remove the last half of the log string. Change this logic if you wish to maintain more/less of the information in the System Status string."
        # "Update System Status - Add a new string to the beginning of the System Status string on the UI."
        n195 = Variant To Data(error in=w413, type="", Variant=w410) -> (data=w407:string, error out=w411:errorcluster)
        n196 = local read "System Status"() -> (w405:string)
        n197 = global read "Global - Configuration Options.vi" "Error Log Max Size (bytes)"() -> (w403:i64)
        n198 = String Length(string=w405) -> (length=w406:i32)
        n199 = Greater?(x=w406, y=w403) -> (0:w404:bool)
        n200 = case shown="True" w404 {
          tunnel: w405 -> [w414 w418]
          tunnel: w403 -> [_ w417]
          tunnel: [w414 w419] -> w402
          frame False {
          }
          frame True {
            n201 = Divide(x=w417, y=i64 2) -> (x/y=w416:dbl)
            n202 = String Subset(string=w418, length (rest)=w416) -> (substring=w419:string)  [unwired: 1 in]
          }
        }
        n203 = Concatenate Strings(w407, w402) -> (→"System Status":string)
      }
      frame "Exit" {
        # "Close all connections"
        # "Stop Monitoring Loop"
        # "Stop Event Handling Loop"
        # "Release the UI Message queue reference"
        # "Stop UI Message Loop"
        # "Exit - Fire the User Event to stop the Event Handling Loop, and toggle the local variable to stop the Monitoring Loop.  This message alone causes all three loops to stop."
        n204 = global write "Global - All UI Loop Stop.vi" "All UI Loop Stop"(TRUE ("Stop Monitoring Loop")) -> ()
        n205 = call "Fire User Event - Stop.vi"("User Event - Stop"=w428) -> ("error out"=w427:errorcluster)  [unwired: 10 in]
        n206 = Release Queue(queue=w424, error in (no error)=w429) -> (error out=w425:errorcluster)  [unwired: 1 in, 2 out]
        n207 = global read "Global - UI Stream and Variable Connections.vi" "UI Command Stream"() -> (w422:refnum<k21>)
        n208 = global read "Global - UI Stream and Variable Connections.vi" "RT Message Stream"() -> (w421:refnum<k21>)
        n209 = global read "Global - UI Stream and Variable Connections.vi" "Variable References"() -> (w420:T9)
        n210 = Destroy Stream Endpoint(11:w422) -> ()  [unwired: 1 in, 1 out]
        n211 = Destroy Stream Endpoint(11:w421) -> ()  [unwired: 1 in, 1 out]
        n212 = call "Close Variable Connections.vi"("Variable References"=w420) -> ()  [unwired: 11 in]
        n213 = Merge Errors(w427, w425) -> (w430:errorcluster)
      }
      frame "---Copy This Frame---" {
        # "Duplicate this frame when creating new messages.  Change this comment in the duplicated frame to describe this message."
        n214 = Merge Errors(w434) -> (w433:errorcluster)
      }
      frame Default {
        # "'Default' case only runs if there is a message that isn't defined in any of the other cases.  Output a programming error."
        n215 = Format Into String(format string="The invalid message string \"%s\" was received in the Message Handling Loop." ("Invalid Message Loop Message"), w439) -> (resulting string=w436:string)  [unwired: 2 in, 1 out]
        n216 = call <vilib>:"Error Cluster From Error Code.vi"("error message (\"\")"=w436, "error code (0)"=1) -> ("error out"=w437:errorcluster)  [unwired: 7 in]
      }
    }
    n217 = call "UI Error Handler - Message Handler.vi"("error in (no error)"=w135, "Message Queue"=w136) -> ()  [unwired: 9 in, 1 out]
    n218 = call <vilib>:"Clear Errors.vi"("error in (no error)"=w135) -> ("error out"=w134:errorcluster)  [unwired: 6 in]
  }
  n219 = while {
    tunnel: w8 -> [w460]
    shift-right: [w453] -> _
    shift-left: dbl[] [] -> [w452]
    shift-right: [w451] -> _
    shift-left: dbl[] [] -> [w448]
    shift-right: [w450] -> _
    shift-left: dbl[] [] -> [w449]
    shift-right: [w447] -> _
    shift-left: dbl[] [] -> [w444]
    shift-right: [w446] -> _
    shift-left: dbl[] [] -> [w443]
    shift-right: [w445] -> _
    shift-left: dbl[] [] -> [w442]
    stop <- w461 stop-if-true
    # "Only read monitoring variables if:\n1.The UI Main VI is \nconnected to the RT target\nAND\n2. The Pause button is not depressed\nAND\n3. The Save button is not depressed"
    # "Only the 'Exit' message in the UI Message Loop can stop the Monitoring Loop."
    # "Monitoring Loop"
    n220 = local read "Connected?"() -> (w458:bool)
    n221 = Not(x="Pause Button") -> (.not. x?=w455:bool)
    n222 = Divide(x=1000.0, y="Display frequency (Hz)") -> (x/y=w441:dbl)
    n223 = And(x=w458, y=w455) -> (x .and. y?=w456:bool)
    n224 = case shown="True" w456 {
      tunnel: w460 -> [_ w579]
      tunnel: w441 -> [w476 w574]
      tunnel: [w473 w513] -> w453
      tunnel: w452 -> [w472 w569]
      tunnel: [w468 w511] -> w451
      tunnel: [w470 w512] -> w450
      tunnel: w449 -> [w471 w563]
      tunnel: w448 -> [w469 w562]
      tunnel: [w466 w510] -> w447
      tunnel: [w464 w509] -> w446
      tunnel: [w462 w508] -> w445
      tunnel: w444 -> [w467 w552]
      tunnel: w443 -> [w465 w551]
      tunnel: w442 -> [w463 w550]
      tunnel: w441 -> [_ w541]
      frame False {
        n225 = Wait (ms)(milliseconds to wait=w476) -> ()  [unwired: 1 out]
        n226 = Not(x="Clear Button") -> (.not. x?=w474:bool)
        n227 = case shown="False" w474 {
          tunnel: [w488 w501] -> w473
          tunnel: w472 -> [w487 w501]
          tunnel: w471 -> [w486 w500]
          tunnel: [w485 w500] -> w470
          tunnel: w469 -> [w484 w499]
          tunnel: [w483 w499] -> w468
          tunnel: w467 -> [w482 w498]
          tunnel: [w481 w498] -> w466
          tunnel: w465 -> [w480 w497]
          tunnel: [w479 w497] -> w464
          tunnel: w463 -> [w478 w496]
          tunnel: [w477 w496] -> w462
          frame False {
            n228 = stacked-sequence {
              tunnel: [dbl[] [] _] -> w488
              tunnel: w487 -> [_ _]
              tunnel: w486 -> [_ _]
              tunnel: [dbl[] [] _] -> w485
              tunnel: w484 -> [_ _]
              tunnel: [dbl[] [] _] -> w483
              tunnel: w482 -> [_ _]
              tunnel: [dbl[] [] _] -> w481
              tunnel: w480 -> [_ _]
              tunnel: [dbl[] [] _] -> w479
              tunnel: w478 -> [_ _]
              tunnel: [dbl[] [] _] -> w477
              frame #0 {
                # "Clear all arrays"
              }
              frame #1 {
                w495 = FALSE ("Clear Button")
                n229 = local write "Pause Button"(w495) -> ()
                n230 = local write "Clear Button"(w495) -> ()
              }
            }
          }
          frame True {
          }
        }
      }
      frame True {
        # "Build the array for plotting"
        # "Get the time data"
        # "Serialize the shared variable calls to simplify the scheduling performed by LabVIEW at runtime"
        n231 = global read "Global - UI Stream and Variable Connections.vi" "Variable References"() -> (w577:T9)
        n232 = call "UI - Read Stream from RT.vi"("Message Queue"=w579) -> ("error out"=w585:errorcluster, "Message Received?"=w575:bool, "dup Message Queue"=w578:refnum<queue>)  [unwired: 8 in]
        n233 = case shown="False" w575 {
          tunnel: w574 -> [w631 _]
          frame False {
            n234 = Wait (ms)(milliseconds to wait=w631) -> ()  [unwired: 1 out]
          }
          frame True {
            # "If a message was received, immediately read again"
          }
        }
        n235 = Unbundle By Name(w577) -> ("CPU Usage"=w592:refnum<k21>, "Contiguous Memory"=w591:refnum<k21>, "Input Values"=w590:refnum<k21>, "Output Values"=w589:refnum<k21>, "FPGA Mode"=w588:refnum<k21>, "Actual Loop Period"=w587:refnum<k21>)
        n236 = Divide(x=w541, y=2.0) -> (x/y=w521:dbl)
        n237 = shared-variable-read(w592, w585) -> (w584:errorcluster, →"CPU Usage (%)":dbl)  [unwired: 2 out]
        n238 = shared-variable-read(w591, w584) -> (w583:errorcluster, →"Largest Contiguous Memory (bytes)":dbl)  [unwired: 2 out]
        n239 = shared-variable-read(w590, w583) -> (w582:errorcluster, w594:T10)  [unwired: 2 out]
        n240 = shared-variable-read(w589, w582) -> (w581:errorcluster, w593:T10)  [unwired: 2 out]
        n241 = shared-variable-read(w588, w581) -> (w580:errorcluster, →"Current FPGA Control Mode":T14)  [unwired: 2 out]
        n242 = shared-variable-read(w587, w580) -> (w586:errorcluster, w540:u32)  [unwired: 2 out]
        "Actual Loop Period (ticks)" <- w540
        n243 = To Double Precision Float(number=w594) -> (double precision float=w573:T11)
        n244 = To Double Precision Float(number=w593) -> (double precision float=w597:T11)
        n245 = Unbundle By Name(w597) -> ("Channel 0"=w561:dbl, "Channel 1"=w559:dbl, "Channel 2"=w557:dbl)
        n246 = Unbundle By Name(w573) -> ("Channel 0"=w547:dbl, "Channel 1"=w566:dbl)
        n247 = Get Date/Time In Seconds() -> (seconds since 1Jan1904=w570:timestamp)
        n248 = Multiply(x=1000.0, y=w547) -> (x*y=w546:dbl)
        n249 = To Double Precision Float(number=w570) -> (double precision float=w549:dbl)
        n250 = Build Array(w546) -> (w564:dbl[])
        n251 = Build Array(w566) -> (w565:dbl[])
        n252 = Build Array(w561) -> (w560:dbl[])
        n253 = Build Array(w559) -> (w558:dbl[])
        n254 = Build Array(w557) -> (w556:dbl[])
        n255 = Build Array (concatenate)(w569, w549) -> (w519:dbl[])
        n256 = Build Array (concatenate)(w563, w564) -> (w524:dbl[])
        n257 = Build Array (concatenate)(w562, w565) -> (w527:dbl[])
        n258 = Build Array (concatenate)(w552, w560) -> (w530:dbl[])
        n259 = Build Array (concatenate)(w551, w558) -> (w533:dbl[])
        n260 = Build Array (concatenate)(w550, w556) -> (w536:dbl[])
        n261 = Divide(x=u32 40000000, y=w540) -> (x/y=→"Control loop frequency (Hz)":dbl)
        n262 = call "Convert to Dynamic Data2"("Array"=w527) -> ("Dynamic Data Type"=w526:dynamicdata)  [unwired: 3 in]
        n263 = call "Convert to Dynamic Data6"("Array"=w536) -> ("Dynamic Data Type"=w535:dynamicdata)  [unwired: 3 in]
        n264 = call "Convert to Dynamic Data3"("Array"=w530) -> ("Dynamic Data Type"=w529:dynamicdata)  [unwired: 3 in]
        n265 = call "Convert to Dynamic Data4"("Array"=w533) -> ("Dynamic Data Type"=w532:dynamicdata)  [unwired: 3 in]
        n266 = call "Convert to Dynamic Data"("Array"=w524) -> ("Dynamic Data Type"=w523:dynamicdata)  [unwired: 3 in]
        n267 = call "Filter"("Lower Cut-Off"=w521, "Signal"=w526) -> ("Filtered Signal"=w525:dynamicdata)  [unwired: 8 in, 1 out]
        n268 = call "Filter"("Lower Cut-Off"=w521, "Signal"=w535) -> ("Filtered Signal"=w534:dynamicdata)  [unwired: 8 in, 1 out]
        n269 = call "Filter"("Lower Cut-Off"=w521, "Signal"=w529) -> ("Filtered Signal"=w528:dynamicdata)  [unwired: 8 in, 1 out]
        n270 = call "Filter"("Lower Cut-Off"=w521, "Signal"=w532) -> ("Filtered Signal"=w531:dynamicdata)  [unwired: 8 in, 1 out]
        n271 = call "Filter"("Lower Cut-Off"=w521, "Signal"=w523) -> ("Filtered Signal"=w522:dynamicdata)  [unwired: 8 in, 1 out]
        n272 = call "Convert from Dynamic Data2"("Dynamic Data Type"=w525) -> ("Array"=w517:dbl[])  [unwired: 3 in]
        n273 = call "Convert from Dynamic Data6"("Dynamic Data Type"=w534) -> ("Array"=w514:dbl[])  [unwired: 3 in]
        n274 = call "Convert from Dynamic Data3"("Dynamic Data Type"=w528) -> ("Array"=w516:dbl[])  [unwired: 3 in]
        n275 = call "Convert from Dynamic Data4"("Dynamic Data Type"=w531) -> ("Array"=w515:dbl[])  [unwired: 3 in]
        n276 = call "Convert from Dynamic Data"("Dynamic Data Type"=w522) -> ("Array"=w518:dbl[])  [unwired: 3 in]
        n277 = Array Size(array=w519) -> (size(s)=w571:i32)
        n278 = Greater?(x=w571, y="Number of points") -> (0:w572:bool)
        n279 = case shown="True" w572 {
          tunnel: w518 -> [w614 w627]
          tunnel: w519 -> [w615 w629]
          tunnel: w571 -> [_ w630]
          tunnel: "Number of points" -> [_ w616]
          tunnel: [w615 w628] -> w507
          tunnel: [w614 w626] -> w506
          tunnel: w517 -> [w613 w624]
          tunnel: [w613 w625] -> w505
          tunnel: [w610 w623] -> w504
          tunnel: [w612 w622] -> w503
          tunnel: [w611 w621] -> w502
          tunnel: w516 -> [w610 w620]
          tunnel: w515 -> [w612 w619]
          tunnel: w514 -> [w611 w618]
          frame False {
          }
          frame True {
            n280 = Subtract(x=w630, y=w616) -> (x-y=w617:i32)
            n281 = Array Subset(array=w629, index=w617, length=w616) -> (w628:dbl[])
            n282 = Array Subset(array=w627, index=w617, length=w616) -> (w626:dbl[])
            n283 = Array Subset(array=w624, index=w617, length=w616) -> (w625:dbl[])
            n284 = Array Subset(array=w620, index=w617, length=w616) -> (w623:dbl[])
            n285 = Array Subset(array=w619, index=w617, length=w616) -> (w622:dbl[])
            n286 = Array Subset(array=w618, index=w617, length=w616) -> (w621:dbl[])
          }
        }
        n287 = case shown="False" "Retain data" {
          tunnel: w519 -> [_ w609]
          tunnel: w518 -> [_ w608]
          tunnel: w517 -> [_ w607]
          tunnel: w516 -> [_ w606]
          tunnel: w515 -> [_ w605]
          tunnel: w514 -> [_ w604]
          tunnel: [w598 w609] -> w513
          tunnel: [w599 w608] -> w512
          tunnel: [w600 w607] -> w511
          tunnel: [w601 w606] -> w510
          tunnel: [w602 w605] -> w509
          tunnel: [w603 w604] -> w508
          tunnel: w507 -> [w598 _]
          tunnel: w506 -> [w599 _]
          tunnel: w505 -> [w600 _]
          tunnel: w504 -> [w601 _]
          tunnel: w503 -> [w602 _]
          tunnel: w502 -> [w603 _]
          frame False {
          }
          frame True {
          }
        }
        n288 = call <vilib>:"Std Deviation and Variance.vi"("X"=w503) -> ("mean"=→"F avg":dbl, "standard deviation"=→"F std":dbl)  [unwired: 1 in, 1 out]
        n289 = Bundle(w507, "Array"=w506) -> (w568:cluster{dbl[], "Array":dbl[]})  [unwired: 1 in]
        n290 = Bundle(w507, "Array"=w505) -> (w567:cluster{dbl[], "Array":dbl[]})  [unwired: 1 in]
        n291 = Bundle(w507, "Array"=w503) -> (→"Force (N)":cluster{dbl[], "Array":dbl[]})  [unwired: 1 in]
        n292 = Bundle(w507, "Array"=w504) -> (→"V*":cluster{dbl[], "Array":dbl[]})  [unwired: 1 in]
        n293 = Bundle(w507, "Array"=w502) -> (→"Position (mm)":cluster{dbl[], "Array":dbl[]})  [unwired: 1 in]
        n294 = Build Array(w568, w567) -> (→"Inputs (mV or V)":cluster{dbl[], "Array":dbl[]}[])
        n295 = call "UI Error Handler - Monitoring.vi"("error in (no error)"=w586, "Message Queue"=w578) -> ()  [unwired: 9 in, 1 out]
      }
    }
    n296 = global read "Global - All UI Loop Stop.vi" "All UI Loop Stop"() -> (w461:bool)
  }
  n297 = Unregister For Events(event registration refnum=w11, error in=w19) -> (error out=w12:errorcluster)
  n298 = Merge Errors(w12, w20) -> (w18:errorcluster)
  n299 = call "Destroy User Event - Stop.vi"("error in (no error)"=w18, "User Event - Stop"=w16) -> ("error out"=w9:errorcluster)  [unwired: 9 in]
  n300 = call <vilib>:"Simple Error Handler.vi"("error in (no error)"=w9) -> ()  [unwired: 4 in, 5 out]
